vi "GlobalImagingStatus.vi"() -> ()   [LabVIEW 2019, in "Global.lvlib"]
uses:
  Global.lvlib
  controls/ImagingStatusControl.ctl
panel:
  in  "ImagingStatus":T1=enum."PMT"
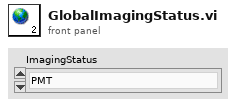
[diagram p1: front panel]
types:
  T1 = typedef "ImagingStatusControl.ctl" = enum16{"PMT_large", "Camera_large", "PMT", "Camera", "Idle"}
diagram:
